vi "regBoxnCube.vi"() -> (0 "BoxColor":u32, 1 "BoxString":string, 2 "CubeColor":u32, 3 "CubeString":string)   [LabVIEW 2017]
uses:
  GlobalVariable.vi
panel:
  out "colorBoxArray":dbl[](array[numeric])
  out "size(box)":i32
  out "colorCubeArray":dbl[](array[numeric])
  out "boxOrange":i32
  out "boxBlue":i32
  out "boxRed":i32
  out "boxYellow":i32
  out "boxGreen":i32
  out "Box is Orange":bool
  out "Box is blue":bool
  out "Box is red":bool
  out "Box is yellow":bool
  out "Box is green":bool
  out "size(cube)":i32
  out "Time has Elapsed":bool
  out "Elapsed Time (s)":dbl
  out "cube is orange":bool
  out "cube is blue":bool
  out "cube is red":bool
  out "cube is yellow":bool
  out "cube is green":bool
  out "cubeOrange":i32
  out "cubeBlue":i32
  out "cubeRed":i32
  out "cubeYellow":i32
  out "cubeGreen":i32
  out "Image Out":T1(plugin-control)
  # "with camera setting \nBightness 148\nContrast 30\nSaturation 40\nSharpness 175"
  # "0 green\n1 yellow\n2 red\n3 blue\n4 orange"
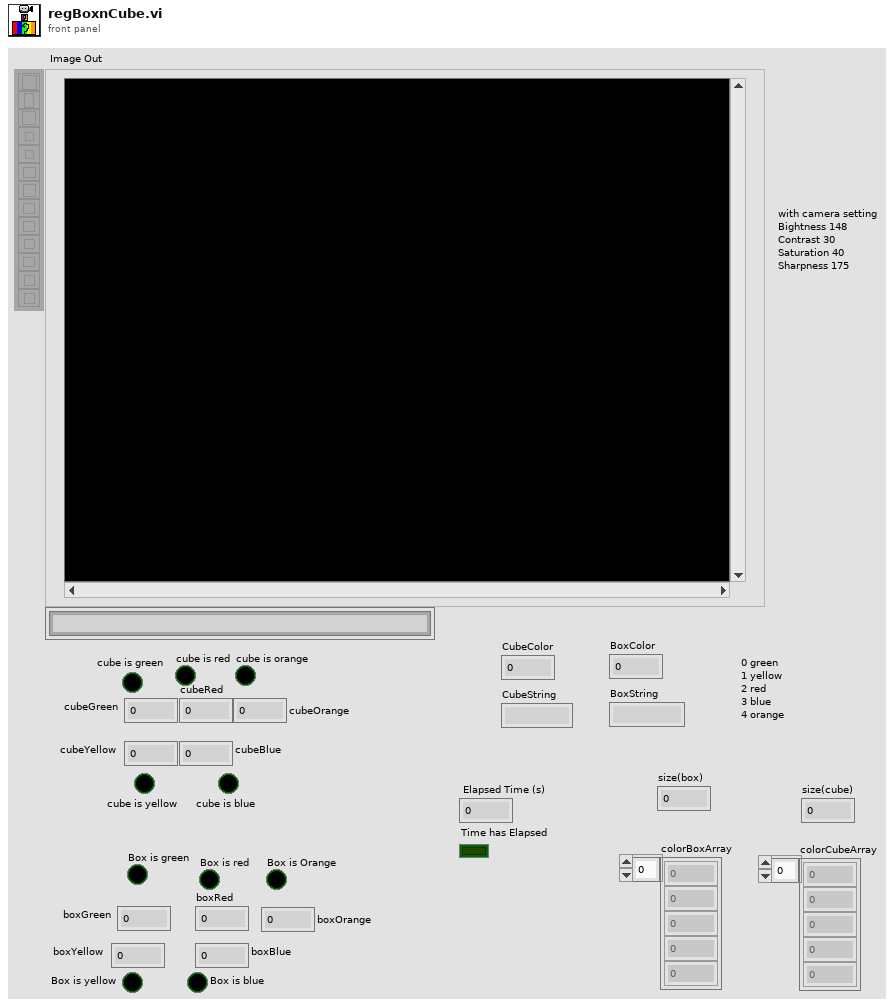
[diagram p1: front panel]
types:
  T1 = typedef "IMAQ Image.ctl" = refnum<image>
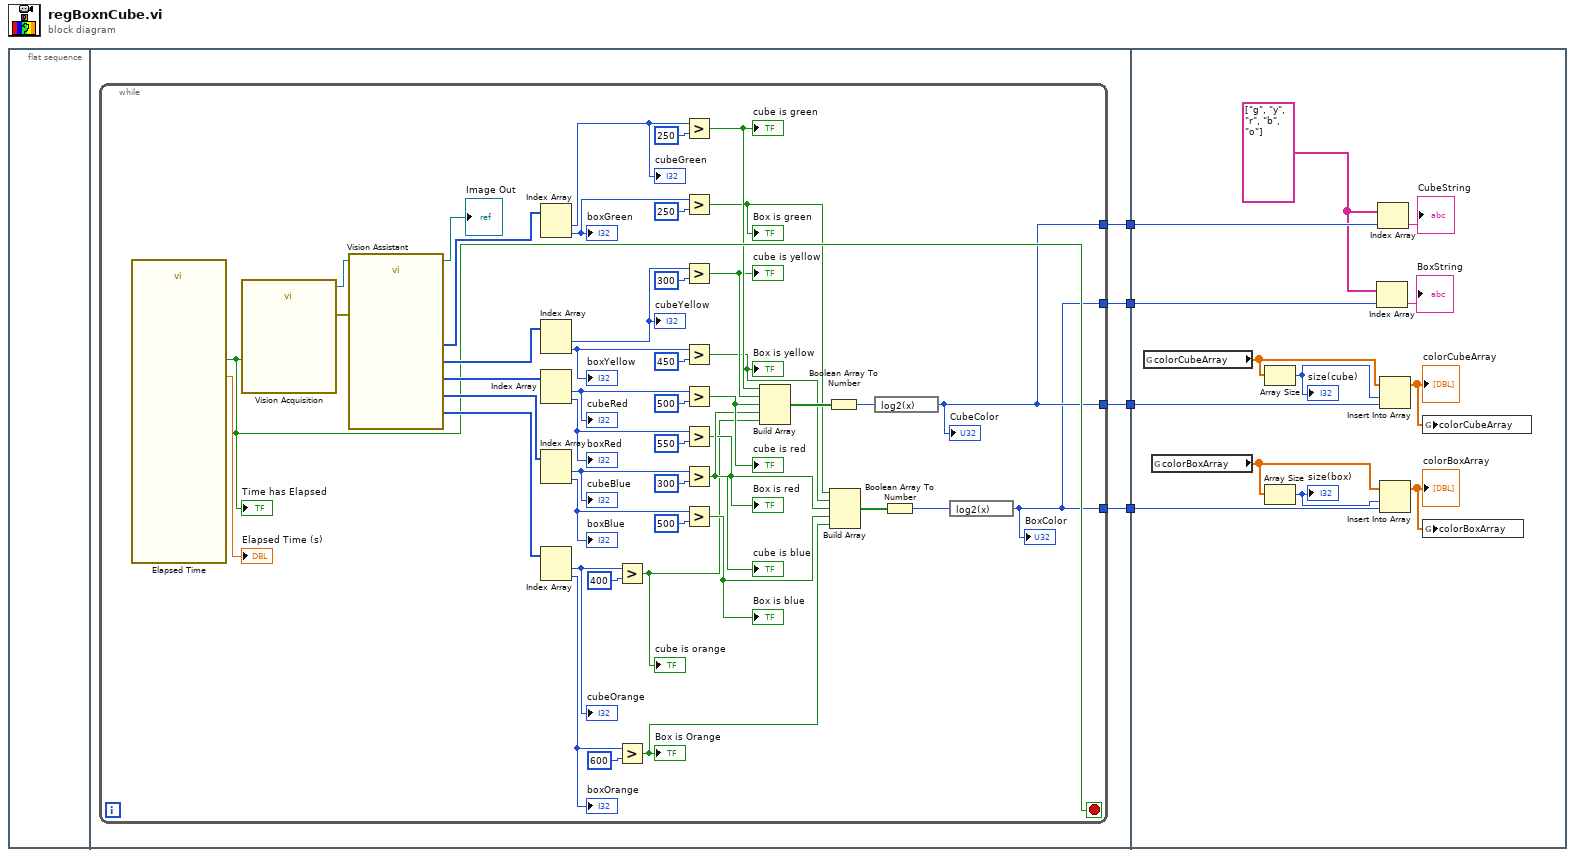
[diagram p0: block diagram]
diagram:
  n1 = flat-sequence {
    tunnel: [w8] -> w4
    tunnel: [w7] -> w3
    tunnel: [w6] -> w2
    tunnel: [w5] -> w1
    tunnel: w4 -> [w65]
    tunnel: w3 -> [w60]
    tunnel: w2 -> [w59]
    tunnel: w1 -> [w56]
    frame #0 {
    }
    frame #1 {
      n2 = while {
        tunnel: [w10] -> w8
        tunnel: [w9] -> w7
        tunnel: [w10] -> w6
        tunnel: [w9] -> w5
        stop <- w35 stop-if-true
        n3 = call "Elapsed Time"() -> ("Elapsed Time (s)"=→"Elapsed Time (s)":dbl, "Time has Elapsed"=w35:bool)  [unwired: 12 in, 6 out]
        "Time has Elapsed" <- w35
        n4 = call "Vision Acquisition"("Stop (F)"=w35) -> ("Image Out"=w53:T1, "error out"=w54:errorcluster)  [unwired: 24 in, 1 out]
        n5 = call "Vision Assistant"("Image In"=w53, "error in"=w54) -> ("Image Out"=→"Image Out":T1, "Match Score (green)"=w51:i32[], "Match Score (yellow)"=w50:i32[], "Match Score (red)"=w49:i32[], "Match Score (blue)"=w48:i32[], "Match Score (orange)"=w47:i32[])  [unwired: 19 in, 1 out]
        n6 = Index Array(array=w51) -> (element #1=w46:i32, element #2=w16:i32)  [unwired: 2 in]
        "cubeGreen" <- w46
        "boxGreen" <- w16
        n7 = Index Array(array=w50) -> (element #1=w44:i32, element #2=w15:i32)  [unwired: 2 in]
        "cubeYellow" <- w44
        "boxYellow" <- w15
        n8 = Index Array(array=w49) -> (element #1=w41:i32, element #2=w14:i32)  [unwired: 2 in]
        "cubeRed" <- w41
        "boxRed" <- w14
        n9 = Index Array(array=w48) -> (element #1=w39:i32, element #2=w13:i32)  [unwired: 2 in]
        "cubeBlue" <- w39
        "boxBlue" <- w13
        n10 = Index Array(array=w47) -> (element #1=w37:i32, element #2=w12:i32)  [unwired: 2 in]
        "cubeOrange" <- w37
        "boxOrange" <- w12
        n11 = Greater?(x=w37, y=400) -> (0:w11:bool)
        "cube is orange" <- w11
        n12 = Greater?(x=w12, y=600) -> (0:w21:bool)
        "Box is Orange" <- w21
        n13 = Greater?(x=w46, y=250) -> (0:w34:bool)
        "cube is green" <- w34
        n14 = Greater?(x=w16, y=250) -> (0:w23:bool)
        "Box is green" <- w23
        n15 = Greater?(x=w44, y=300) -> (0:w33:bool)
        "cube is yellow" <- w33
        n16 = Greater?(x=w15, y=450) -> (0:w22:bool)
        "Box is yellow" <- w22
        n17 = Greater?(x=w41, y=500) -> (0:w32:bool)
        "cube is red" <- w32
        n18 = Greater?(x=w14, y=550) -> (0:w17:bool)
        "Box is red" <- w17
        n19 = Greater?(x=w39, y=300) -> (0:w31:bool)
        "cube is blue" <- w31
        n20 = Greater?(x=w13, y=500) -> (0:w18:bool)
        "Box is blue" <- w18
        n21 = Build Array(w34, w33, w32, w31, w11) -> (w30:bool[])
        n22 = Boolean Array To Number(Boolean array=w30) -> (number=w29:u32)
        n23 = Build Array(w23, w22, w17, w18, w21) -> (w19:bool[])
        n24 = expression code="log2(x)"(w29) -> (w10:u32)
        "CubeColor" <- w10
        n25 = Boolean Array To Number(Boolean array=w19) -> (number=w20:u32)
        n26 = expression code="log2(x)"(w20) -> (w9:u32)
        "BoxColor" <- w9
      }
    }
    frame #2 {
      w55 = string[] ["g", "y", "r", "b", "o"]
      n27 = global read "GlobalVariable.vi" "colorCubeArray"() -> (w67:dbl[])
      n28 = global read "GlobalVariable.vi" "colorBoxArray"() -> (w63:dbl[])
      n29 = Array Size(array=w67) -> (size(s)=w66:i32)
      "size(cube)" <- w66
      n30 = Array Size(array=w63) -> (size(s)=w62:i32)
      "size(box)" <- w62
      n31 = Index Array(array=w55, index=w56) -> (element=→"BoxString":string)
      n32 = Index Array(array=w55, index=w59) -> (element=→"CubeString":string)
      n33 = Insert Into Array(array=w67, index=w66, new element=w65) -> (w64:dbl[])
      "colorCubeArray" <- w64
      n34 = Insert Into Array(array=w63, index=w62, new element=w60) -> (w61:dbl[])
      "colorBoxArray" <- w61
      n35 = global write "GlobalVariable.vi" "colorCubeArray"(w64) -> ()
      n36 = global write "GlobalVariable.vi" "colorBoxArray"(w61) -> ()
    }
  }
